vi "fmt_reallocateFormatBuffer.vi"(8 "error in (no error)":errorcluster, 10 "Formatted data length":i32, 11 "Format buffers in":T1) -> (0 "error out":errorcluster, 3 "Format buffers out":T1)   [LabVIEW 2017, in "NI_ExcelFile.lvlib"]
uses:
  <vilib>/express/express shared/NI_ExcelFile/NI_ExcelFile.lvlib
  <vilib>/express/express shared/NI_ExcelFile/Ctrls/fmt_formatBuffer.ctl
  <vilib>/express/express shared/NI_ExcelFile/Ctrls/TimeColumnMode.ctl
  <vilib>/express/express shared/NI_ExcelFile/Ctrls/Columns.ctl
  <vilib>/express/express shared/NI_ExcelFile/Ctrls/ColumnInfo.ctl
  <vilib>/express/express shared/NI_ExcelFile/Ctrls/DataType.ctl
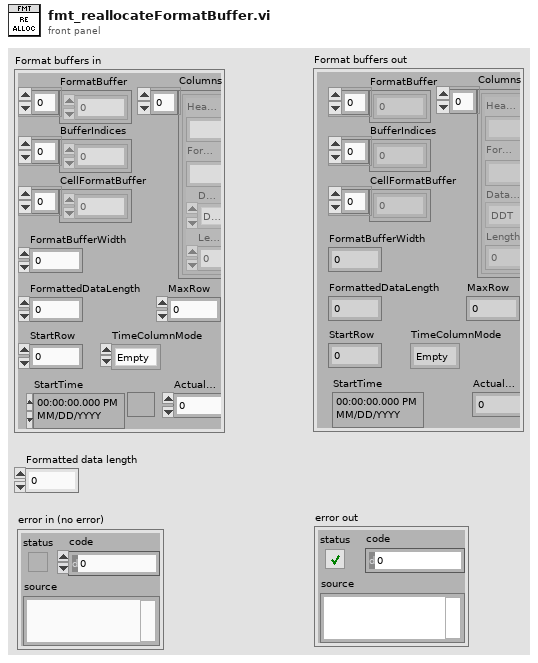
[diagram p1: front panel]
types:
  T1 = typedef "NI_ExcelFile.lvlib/fmt_formatBuffer.ctl" = cluster{"FormatBuffer":u8[], "BufferIndices":i32[], "CellFormatBuffer":u8[], "FormatBufferWidth":i32, "FormattedDataLength":i32, "MaxRow":i32, "StartRow":i32, "TimeColumnMode":T2, "StartTime":timestamp, "Columns":T3, "ActualLength":i32}
  T2 = typedef "NI_ExcelFile.lvlib/TimeColumnMode.ctl" = enum16{"Empty", "OnePerCh", "One"}
  T3 = typedef "NI_ExcelFile.lvlib/Columns.ctl" = T4[]
  T4 = typedef "NI_ExcelFile.lvlib/ColumnInfo.ctl" = cluster{"Header":string, "Format":string, "DataType":T5, "Length":u64}
  T5 = typedef "NI_ExcelFile.lvlib/DataType.ctl" = enum16{"DDT", "WFM", "Array of STR", "Array of DBL", "Array of I8", "Array of I16", "Array of I32", "Array of I64", "Array of SGL", "Array of U8", "Array of U16", "Array of U32", "Array of U64", "Array of Time"}
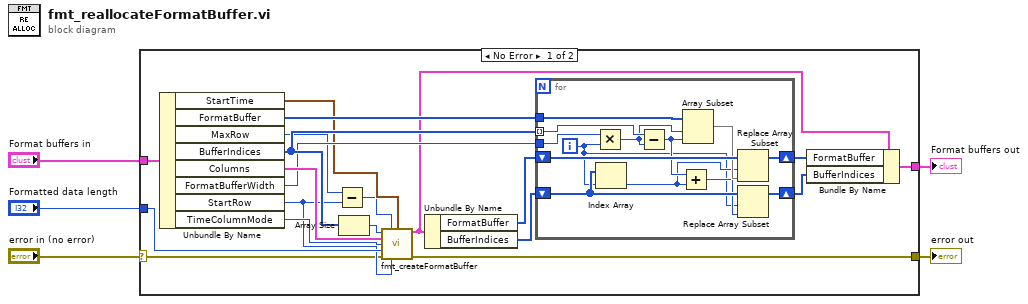
[diagram p0: block diagram]
diagram:
  n1 = case shown="No Error" "error in (no error)" {
    selector: "error in (no error)" -> [w6 w39]
    tunnel: "Format buffers in" -> [w25 w40]
    tunnel: [w17 w40] -> w4
    tunnel: "Formatted data length" -> [w13 _]
    tunnel: [w12 w39] -> w2
    frame No Error {
      n2 = Unbundle By Name(w25) -> ("StartTime"=w10:timestamp, "FormatBuffer"=w21:u8[], "MaxRow"=w9:i32, "BufferIndices"=w22:i32[], "Columns"=w24:T3, "FormatBufferWidth"=w20:i32, "StartRow"=w8:i32, "TimeColumnMode"=w11:T2)
      n3 = Subtract(x=w9, y=w8) -> (x-y=w7:i32)
      n4 = Array Size(array=w22) -> (size(s)=w23:i32)
      n5 = call <vilib>:"fmt_createFormatBuffer.vi"("rows"=w23, "max rows"=w7, "start time"=w10, "columns"=w24, "time column mode"=w11, "predifed formatted value length"=w13, "error in (no error)"=w6, "start row"=w8) -> ("Format buffers out"=w16:T1, "error out"=w12:errorcluster)  [unwired: 6 in]
      n6 = Unbundle By Name(w16) -> ("FormatBuffer"=w19:u8[], "BufferIndices"=w18:i32[])
      n7 = for {
        tunnel: w22 -> [w34] mode=indexing
        tunnel: w21 -> [w35]
        tunnel: w20 -> [w36]
        shift-right: [w37] -> w15
        shift-left: w19 -> [w38]
        shift-right: [w31] -> w14
        shift-left: w18 -> [w30]
        i -> [w26]
        n8 = Multiply(x=w36, y=w26) -> (x*y=w33:i32)
        n9 = Index Array(array=w30, index=w26) -> (element=w28:i32)
        n10 = Subtract(x=w34, y=w33) -> (x-y=w29:i32)
        n11 = Add(x=w29, y=w28) -> (x+y=w27:i32)
        n12 = Array Subset(array=w35, index=w33, length=w29) -> (w32:u8[])
        n13 = Replace Array Subset(array=w38, new element=w32, index=w28) -> (w37:u8[])
        n14 = Replace Array Subset(array=w30, new element=w27, index=w26) -> (w31:i32[])
      }
      n15 = Bundle By Name(cluster=w16, "FormatBuffer"=w15, "BufferIndices"=w14) -> (w17:T1)
    }
    frame Error {
    }
  }
  "Format buffers out" <- w4
  "error out" <- w2
